vi "Setup Size Data.vi"(8 "Error":errorcluster, 9 "Border Spacing":i16, 11 "FP":refnum<class "DecFrame_FP.lvclass">) -> (0 "Error Out":errorcluster, 3 "FP Out":refnum<class "DecFrame_FP.lvclass">)   [LabVIEW 2023, in "DecFrame_FP.lvclass"]
uses:
  DecFrame_FP.lvclass
  DecFrame_FP.lvclass/DecFrame_FP.ctl
  GObject_FPSZ/GObject_FPSZ.lvclass
  FPSZ/FPSZ.lvclass
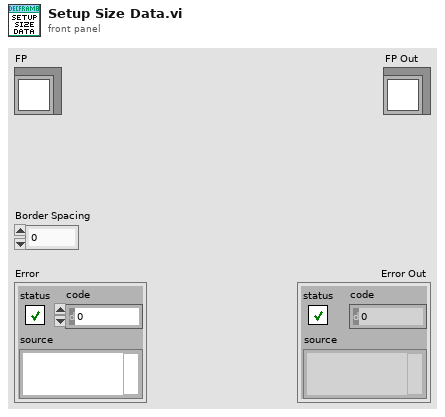
[diagram p1: front panel]
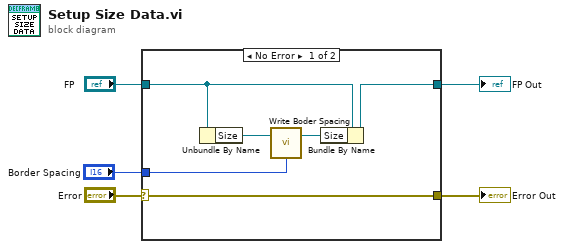
[diagram p0: block diagram]
diagram:
  n1 = case shown="No Error" "Error" {
    selector: "Error" -> [w9 w13]
    tunnel: [w9 w13] -> w4
    tunnel: [w10 w12] -> w2
    tunnel: "FP" -> [w11 w12]
    tunnel: "Border Spacing" -> [w6 _]
    frame No Error {
      n2 = Unbundle By Name(w11) -> ("Size"=w8:refnum<class "GObject_FPSZ.lvclass">)
      n3 = call "Write Boder Spacing.vi"("(FPSZ)"=w8, "Border Spacing"=w6) -> ("(FPSZ) Out"=w7:refnum<class "GObject_FPSZ.lvclass">)  [unwired: 3 in]
      n4 = Bundle By Name(cluster=w11, "Size"=w7) -> (w10:refnum<class "DecFrame_FP.lvclass">)
    }
    frame Error {
    }
  }
  "Error Out" <- w4
  "FP Out" <- w2
